vi "ModifyImage ctab.vi"(4 "maximum":dbl, 6 "minimum":dbl, 8 "error in (no error)":errorcluster, 9 "Invert Color Scheme? [NO]":bool, 10 "Color Table Name [VioletOrangeYellow]":string="Rainbow", 11 "ITX Commands in":refnum<class "ITX Commands.lvclass">) -> (0 "error out":errorcluster, 3 "ITX Commands out":refnum<class "ITX Commands.lvclass">)   [LabVIEW 2019, in "ITX Commands.lvclass"]
uses:
  ITX Commands.lvclass
  ITX Commands.lvclass/ITX Commands.ctl
panel:
  out "resulting string":string="ModifyImage '' ctab{,, Rainbow, 0}"
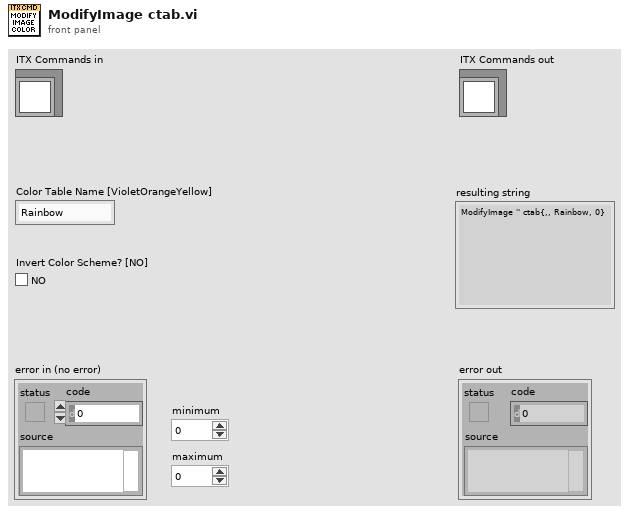
[diagram p1: front panel]
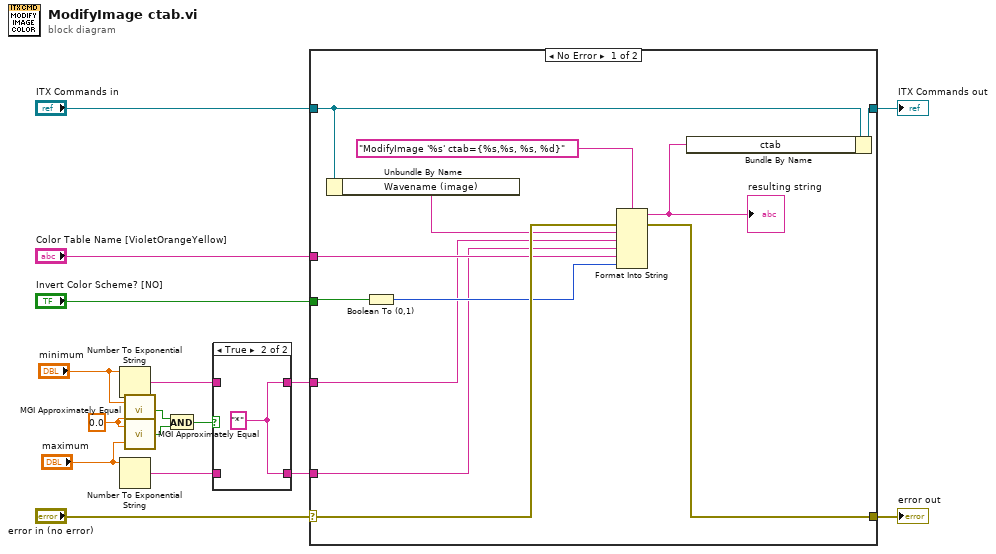
[diagram p0: block diagram]
diagram:
  w3 = 0.0 ("Numeric 2")
  n1 = Number To Exponential String(number="minimum") -> (E-format string=w5:string)  [unwired: 3 in]
  n2 = Number To Exponential String(number="maximum") -> (E-format string=w6:string)  [unwired: 3 in]
  n3 = call <userlib>:"MGI Approximately Equal.vi"("Numeric 2"=w3, "Numeric 1"="minimum") -> ("approx = ?"=w9:bool)
  n4 = call <userlib>:"MGI Approximately Equal.vi"("Numeric 2"="maximum", "Numeric 1"=w3) -> ("approx = ?"=w10:bool)
  n5 = And(x=w9, y=w10) -> (x .and. y?=w4:bool)
  n6 = case shown="True" w4 {
    tunnel: [w18 w19] -> w8
    tunnel: [w17 w19] -> w7
    tunnel: w6 -> [w17 _]
    tunnel: w5 -> [w18 _]
    frame False {
    }
    frame True {
      w19 = "*" ("t")
    }
  }
  n7 = case shown="No Error" "error in (no error)" {
    selector: "error in (no error)" -> [w27 w33]
    tunnel: [w26 w33] -> w15
    tunnel: [w28 w32] -> w13
    tunnel: "ITX Commands in" -> [w29 w32]
    tunnel: "Color Table Name [VioletOrangeYellow]" -> [w23 _]
    tunnel: "Invert Color Scheme? [NO]" -> [w30 _]
    tunnel: w8 -> [w22 _]
    tunnel: w7 -> [w21 _]
    frame No Error {
      n8 = Unbundle By Name(w29) -> ("Wavename (image)"=w25:string)
      n9 = Boolean To (0,1)(Boolean=w30) -> (0, 1=w24:i16)
      n10 = Format Into String(format string="ModifyImage '%s' ctab={%s,%s, %s, %d}", error in=w27, w25, w22, w21, w23, w24) -> (resulting string=w20:string, error out=w26:errorcluster)  [unwired: 1 in]
      "resulting string" <- w20
      n11 = Bundle By Name(cluster=w29, "ctab"=w20) -> (w28:refnum<class "ITX Commands.lvclass">)
    }
    frame Error {
    }
  }
  "error out" <- w15
  "ITX Commands out" <- w13
